vi "Clamp Positions.vi"(1 "Shortest (LS)":bool, 2 "Wide (BB)":bool, 3 "Widest (LS)":bool) -> (0 "Clamp Position":dbl)   [LabVIEW 2014]
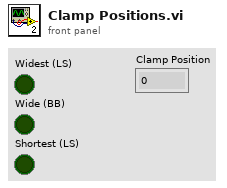
[diagram p1: front panel]
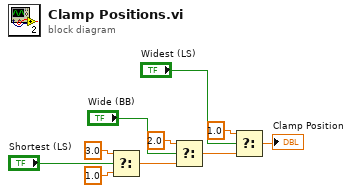
[diagram p0: block diagram]
diagram:
  n1 = Select(t=3.0, s="Shortest (LS)", f=1.0) -> (s? t:f=w1:dbl)
  n2 = Select(t=2.0, s="Wide (BB)", f=w1) -> (s? t:f=w7:dbl)
  n3 = Select(t=1.0, s="Widest (LS)", f=w7) -> (s? t:f=→"Clamp Position":dbl)
